vi "CFTS-Get Data Folder.vi"(5 "Drive":string, 7 "Root folder":path, 8 "error in (no error)":errorcluster, 9 "create?":bool, 10 "Number":i32, 11 "Experimenter":string) -> (0 "error out":errorcluster, 2 "Data folder":path)   [LabVIEW 2020]
doc: "Takes an experiment ID (e.g. KEH999) and returns the standard data folder (e.g. C:\\Data\\KEH DATA\\KEH999)"
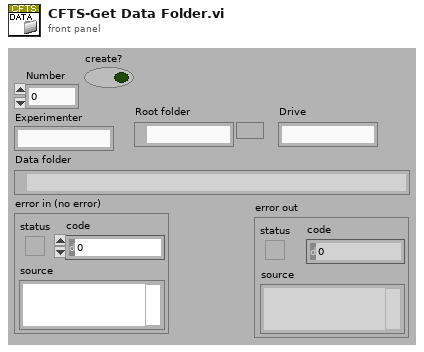
[diagram p1: front panel]
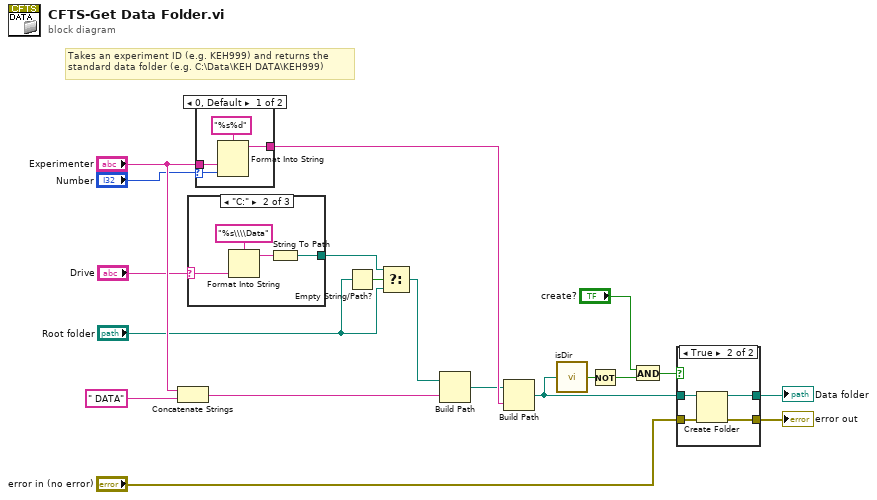
[diagram p0: block diagram]
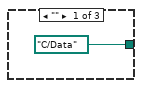
[diagram p2: hidden frame]
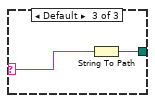
[diagram p3: hidden frame]
diagram:
  # "Takes an experiment ID (e.g. KEH999) and returns the\nstandard data folder (e.g. C:\\Data\\KEH DATA\\KEH999)"
  n1 = Concatenate Strings("Experimenter", " DATA" ("string")) -> (w18:string)
  n2 = case shown="\"C:\"" "Drive" {
    selector: "Drive" -> [_ w23 w25]
    tunnel: [path "C:/Data" ("base path") w21 w26] -> w3
    frame "" {
    }
    frame "C:" {
      n3 = Format Into String(format string="%s\\\\Data", w23) -> (resulting string=w22:string)  [unwired: 2 in, 1 out]
      n4 = String To Path(string=w22) -> (path=w21:path)
    }
    frame Default {
      n5 = String To Path(string=w25) -> (path=w26:path)
    }
  }
  n6 = case shown="0, Default" "Number" {
    selector: "Number" -> [w28 _]
    tunnel: "Experimenter" -> [w29 w31]
    tunnel: [w27 w31] -> w15
    frame 0, Default {
      n7 = Format Into String(format string="%s%d", w29, w28) -> (resulting string=w27:string)  [unwired: 2 in, 1 out]
    }
    frame -1 {
    }
  }
  n8 = Empty String/Path?(string/path="Root folder") -> (empty?=w6:bool)
  n9 = Select(t=w3, s=w6, f="Root folder") -> (s? t:f=w2:path)
  n10 = Build Path(base path=w2, name or relative path=w18) -> (appended path=w1:path)
  n11 = Build Path(base path=w1, name or relative path=w15) -> (appended path=w14:path)
  n12 = call "isDir.vi"("path"=w14) -> ("is Dir?"=w12:bool)
  n13 = Not(x=w12) -> (.not. x?=w10:bool)
  n14 = And(x="create?", y=w10) -> (x .and. y?=w11:bool)
  n15 = case shown="True" w11 {
    tunnel: w14 -> [w33 w37]
    tunnel: "error in (no error)" -> [w32 w36]
    tunnel: [w33 w35] -> w8
    tunnel: [w32 w34] -> w7
    frame False {
    }
    frame True {
      n16 = Create Folder(path (use dialog)=w37, error in=w36) -> (created path=w35:path, error out=w34:errorcluster)  [unwired: 1 in, 1 out]
    }
  }
  "Data folder" <- w8
  "error out" <- w7
